vi "switch_dataOLD.vi"(7 "LabVIEW Web Service Request":refnum<class "Web Request.lvclass">) -> ()   [LabVIEW 2014]
uses:
  <vilib>/wsapi/Web Request.lvclass
  DataManager/StateStore/Controls/DataFunction.ctl
panel:
  # "Use the Web Service Request input terminal to call the VIs on the Web Services palette. Do not remove it from the connector pane unless you don't need access to the palette."
  # "Each additional control wired to the connector pane will be available as an input in the URL. To include an indicator in terminal-mode output (the default setting), it must also be wired to the connector pane."
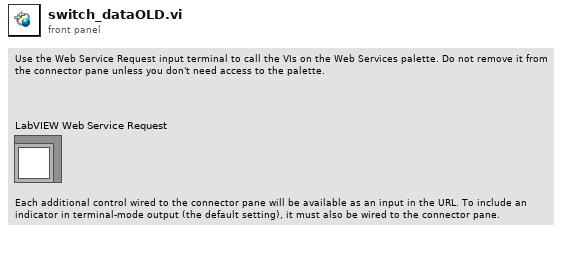
[diagram p1: front panel]
types:
  T1 = cluster{"switch_posit":cluster{"x":dbl, "y":dbl, "z":dbl}, "manual":bool}
  T2 = typedef "DataFunction.ctl" = enum16{"Initialise", "Release", "Get Data", "Set Data", "Preview Data"}
  T3 = typedef "CData Core Control.ctl" = cluster{"train_data_array":cluster{"uuid":string, "int":i32, "posit_array":cluster{"x":dbl, "y":dbl, "z":dbl}[]}[], "train_control_array":cluster{"uuid":string, "throttle":dbl, "brake":dbl, "horn":dbl, "wait":dbl, "name":string, "mode":string, "dest":string}[], "switch_data_array":cluster{"switch_posit":cluster{"x":dbl, "y":dbl, "z":dbl}, "manual":bool}[], "switch_control_array":cluster{"switch_posit":cluster{"x":dbl, "y":dbl, "z":dbl}, "switch":bool, "invert":bool, "wait":dbl}[]}
  T4 = cluster{"switch_posit":cluster{"x":dbl, "y":dbl, "z":dbl}, "manual":bool}[]
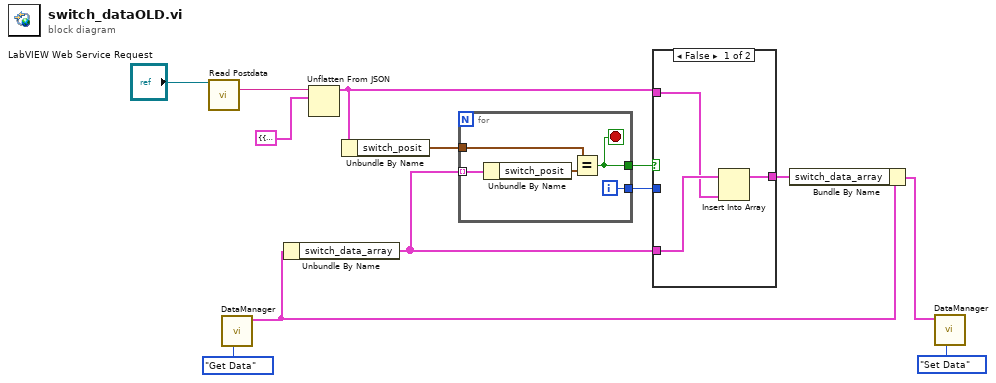
[diagram p0: block diagram]
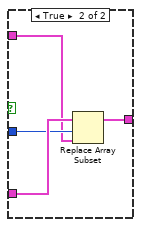
[diagram p2: hidden frame]
diagram:
  n1 = call <vilib>:"Read Postdata.vi"("LabVIEW Web Service Request"="LabVIEW Web Service Request") -> ("postdata"=w9:string)  [unwired: 12 in, 2 out]
  n2 = call "DataManager.vi"("DataFunction"=DataFunction."Get Data") -> ("CData Out"=w8:T3)  [unwired: 9 in, 1 out]
  n3 = Unbundle By Name(w8) -> ("switch_data_array"=w4:T4)
  n4 = Unflatten From JSON(JSON string=w9, type and defaults=T1 {"switch_posit"={"x"=0.0, "y"=0.0, "z"=0.0}, "manual"=FALSE} ("switch_data")) -> (value=w3:T1)  [unwired: 5 in, 1 out]
  n5 = Unbundle By Name(w3) -> ("switch_posit"=w7:cluster{"x":dbl, "y":dbl, "z":dbl})
  n6 = for {
    tunnel: w4 -> [w18] mode=indexing
    tunnel: w7 -> [w16]
    tunnel: [w15] -> w6
    tunnel: [w14] -> w5
    i -> [w14]
    stop <- w15 stop-if-true
    n7 = Unbundle By Name(w18) -> ("switch_posit"=w17:cluster{"x":dbl, "y":dbl, "z":dbl})
    n8 = Equal?(x=w16, y=w17) -> (x = y?=w15:bool)
  }
  n9 = case shown="False" w6 {
    tunnel: w5 -> [_ w24]
    tunnel: w4 -> [w21 w25]
    tunnel: w3 -> [w20 w23]
    tunnel: [w19 w22] -> w2
    frame False {
      n10 = Insert Into Array(array=w21, new element=w20) -> (w19:T4)  [unwired: 1 in]
    }
    frame True {
      n11 = Replace Array Subset(array=w25, new element=w23, index=w24) -> (w22:T4)
    }
  }
  n12 = Bundle By Name(cluster=w8, "switch_data_array"=w2) -> (w11:T3)
  n13 = call "DataManager.vi"("DataFunction"=DataFunction."Set Data", "CData In"=w11) -> ()  [unwired: 8 in, 2 out]
